vi "GetTxDetectorVolts.vi"(3 "error in (no error)":errorcluster) -> (0 "error out":errorcluster, 1 "String_Volts_TxDet":string, 2 "Volts Tx Detector":dbl format="%#.10f")   [LabVIEW 2009]
doc: "Read voltage from RF Detector near transmitter."
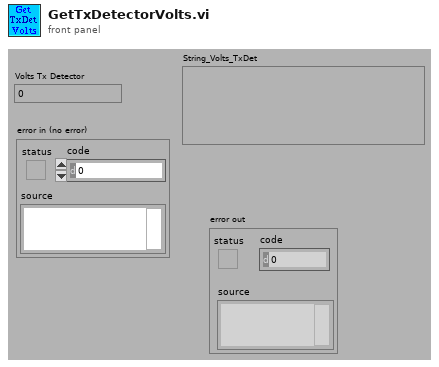
[diagram p1: front panel]
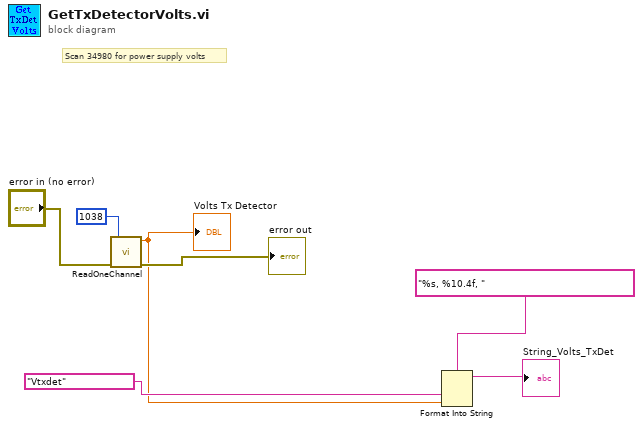
[diagram p0: block diagram]
diagram:
  # "Scan 34980 for power supply volts"
  n1 = call "ReadOneChannel.vi"("error in (no error)"="error in (no error)", "Circuit ID"=1038) -> ("Error out"=→"error out":errorcluster, "OneChannelsValue"=w1:dbl)  [unwired: 4 in]
  "Volts Tx Detector" <- w1
  n2 = Format Into String(format string="%s, %10.4f, ", "Vtxdet", w1) -> (resulting string=→"String_Volts_TxDet":string)  [unwired: 2 in, 1 out]
